vi "Untitled 1.vi"() -> ()   [LabVIEW 2016]
panel:
  in  "x":dbl
  out "error out":errorcluster
  out "Distance 2":dbl
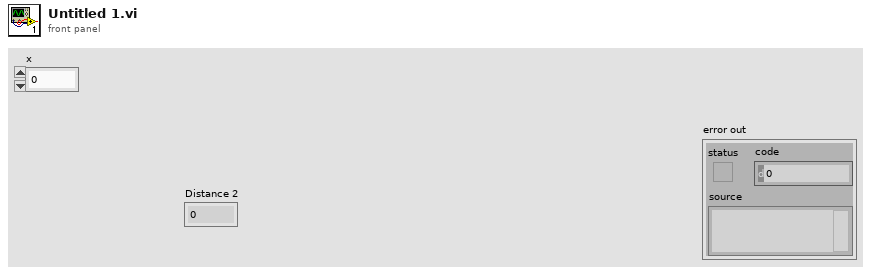
[diagram p1: front panel]
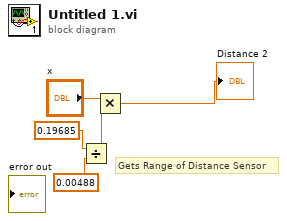
[diagram p0: block diagram]
diagram:
  # "Gets Range of Distance Sensor"
  n1 = Divide(x=0.19685, y=0.00488) -> (x/y=w3:dbl)
  n2 = Multiply(x="x", y=w3) -> (x*y=→"Distance 2":dbl)
